vi "main.vi"() -> ()   [LabVIEW 2015]
uses:
  Program Files/C4Utility/c4hdl/win64-x64/LabVIEW/C4Dev_writeFeature.vi
  Program Files/C4Utility/c4hdl/win64-x64/LabVIEW/libC4HdlLV.lvlib
panel:
  in  "camCfg in":string="# simple configuration example of heliInspect H8 using internal motion control\n#\n# Motion parameters in [mm] or [mm/s]\n# exposure ration between 0.0 and 1.0 [1.0 = 100% exposure]\n#\n# enable required components\nComponentSelector = Intensity\nComponentEnable = false\nComponentSelector = Range\nComponentEnable = true\nComponentSelector = Reflectance\nComponentEnable = true\nComponentSelector = Phase\nComponentEnable = false\n#\n# enable required chunk data (optional)\nChunkModeActive = true\nChunkSelector = PartCount\nChunkEnable = true\nChunkSelector = PartType\nChunkEnable = true\n#\n# trigger configuration\nTriggerSelector = RecordingStart\nTriggerMode = On\nTriggerSource = Stage\nTriggerSelector = AcquisitionStart\nTriggerMode = Off\nTriggerSelector = FrameStart\nTriggerMode = On\nTriggerSource = Software\n# Hint: The TriggerSource also controls the TriggerSoftware feature.\n#\n# encoder configuration\nEncoderSelector = Camera\nEncoderInverter = true\n#\n# motion and position configuration\nScanPosition = -1.4\nScanRange = 0.5\nScanSpeed = 5.0\nGeneralSpeed = 10.0\n#\nScanMode = Down\nStageInit = 1\n#\n# additional camera and processing configuration\nScan3dExtractionMethod = AcceleratedCenterOfMassIQCorrection\nScan3dScalingMethod = zTags\nScan3dDistanceUnit = um\n#\nTargetVerticalSpacing = 2.5\nExposureRatio = 1.0\n#\nFPNCorrection = AverageLastFrames\nFPNCorrectionNFrames = 8\nExtSimpMaxHWin = 7\n#\n# illumination control (D3)\nLightControllerSelector = LightController0\nLightControllerSource = UserOutput0\nLightBrightness = 100.0\n# illumination control (D2)\n# LineSelector = Line2\n# LineSource = UserOutput0\n# LineInverter = True\n# switch on the illumination (D2/D3)\nUserOutputSelector = UserOutput0\nUserOutputValue = true"
  out "acqItr":i32
  out "Surface out":dbl[][](graph)
  out "error out":errorcluster
  out "devName out":string[](array[string])
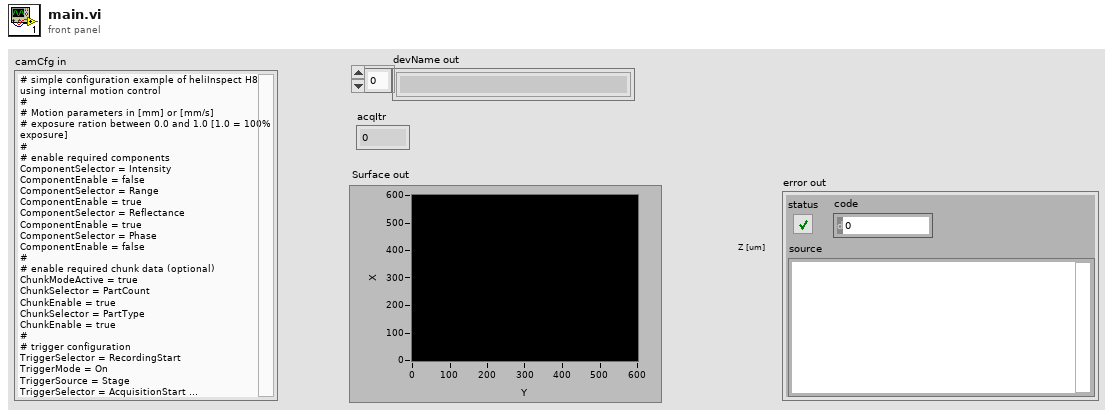
[diagram p1: front panel]
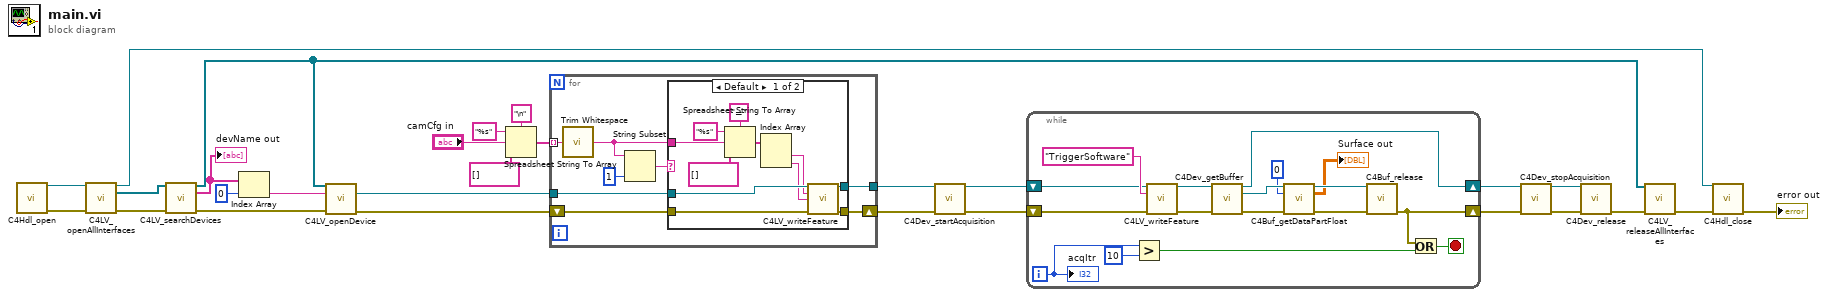
[diagram p0: block diagram]
diagram:
  n1 = call "C4Hdl_open.vi"() -> ("c4hdl out"=w26:refnum<k24>, "error out"=w27:errorcluster)  [unwired: 14 in]
  n2 = call "C4LV_openAllInterfaces.vi"("c4hdl in"=w26, "error in (no error)"=w27) -> ("c4hdl out"=w1:refnum<k24>, "c4if Arr out"=w24:refnum<k24>[], "error out"=w25:errorcluster)  [unwired: 11 in]
  n3 = call "C4LV_searchDevices.vi"("c4if Arr in"=w24, "error in (no error)"=w25) -> ("c4if Arr out"=w11:refnum<k24>[], "devName out"=w23:string[], "error out"=w22:errorcluster)  [unwired: 11 in]
  "devName out" <- w23
  n4 = Index Array(array=w23, index=0) -> (element=w21:string)
  n5 = call "C4LV_openDevice.vi"("c4if Arr in"=w11, "devName in"=w21, "error in (no error)"=w22) -> ("c4dev out"=w20:refnum<k24>, "error out"=w19:errorcluster)  [unwired: 10 in, 1 out]
  n6 = Spreadsheet String To Array(delimiter (Tab)="\n", format string="%s", spreadsheet string="camCfg in", array type (2D Dbl)=string[] [] ("Array Constant")) -> (array=w4:string[])
  n7 = for {
    tunnel: w4 -> [w32] mode=indexing
    tunnel: w20 -> [w33]
    shift-right: [w35] -> w18
    shift-left: w19 -> [w36]
    tunnel: [w34] -> w17
    n8 = call <vilib>:"Trim Whitespace.vi"("string"=w32) -> ("trimmed string"=w31:string)  [unwired: 1 in]
    n9 = String Subset(string=w31, length (rest)=1 ("length (rest)")) -> (substring=w30:string)  [unwired: 1 in]
    n10 = case shown="Default" w30 {
      tunnel: w36 -> [w47 w49]
      tunnel: [w46 w49] -> w35
      tunnel: [w45 w48] -> w34
      tunnel: w33 -> [w44 w48]
      tunnel: w31 -> [w39 _]
      frame Default {
        n11 = Spreadsheet String To Array(delimiter (Tab)="=", format string="%s", spreadsheet string=w39, array type (2D Dbl)=string[] [] ("Array Constant")) -> (array=w43:string[])
        n12 = Index Array(array=w43) -> (element #1=w37:string, element #2=w38:string)  [unwired: 2 in]
        n13 = call-poly "C4LV_writeFeature.vi"("c4dev in"=w44, "name in"=w37, "value in"=w38, "error in"=w47) -> ("c4dev out"=w45:refnum<k24>, "error out"=w46:errorcluster)  [unwired: 10 in]
      }
      frame "#" {
        # "# is a comment"
      }
    }
  }
  n14 = call "C4Dev_startAcquisition.vi"("c4dev in"=w17, "error in (no error)"=w18) -> ("c4dev out"=w16:refnum<k24>, "error out"=w15:errorcluster)  [unwired: 12 in]
  n15 = while {
    shift-right: [w55] -> w10
    shift-left: w15 -> [w56]
    shift-right: [w50] -> w9
    shift-left: w16 -> [w53]
    i -> [w66]
    stop <- w63 stop-if-true
    n16 = Greater?(x=w66, y=10) -> (0:w64:bool)
    n17 = call-poly "C4LV_writeFeature.vi"("c4dev in"=w53, "name in"="TriggerSoftware", "error in"=w56) -> ("c4dev out"=w62:refnum<k24>, "error out"=w57:errorcluster)  [unwired: 11 in]
    n18 = call "C4Dev_getBuffer.vi"("c4dev in"=w62, "error in (no error)"=w57) -> ("c4dev out"=w50:refnum<k24>, "c4buf out"=w60:refnum<k24>, "error out"=w58:errorcluster)  [unwired: 11 in]
    n19 = call "C4Buf_getDataPartFloat.vi"("c4buf in"=w60, "partIdx in"=i64 0, "error in (no error)"=w58) -> ("c4buf out"=w61:refnum<k24>, "data out"=→"Surface out":dbl[][], "error out"=w59:errorcluster)  [unwired: 10 in]
    n20 = call "C4Buf_release.vi"("c4buf in"=w61, "error in (no error)"=w59) -> ("error out"=w55:errorcluster)  [unwired: 13 in]
    n21 = Or(x=w55, y=w64) -> (x .or. y?=w63:bool)
    "acqItr" <- w66
  }
  n22 = call "C4Dev_stopAcquisition.vi"("c4dev in"=w9, "error in (no error)"=w10) -> ("c4dev out"=w13:refnum<k24>, "error out"=w14:errorcluster)  [unwired: 12 in]
  n23 = call "C4Dev_release.vi"("c4dev in"=w13, "error in (no error)"=w14) -> ("error out"=w12:errorcluster)  [unwired: 13 in]
  n24 = call "C4LV_releaseAllInterfaces.vi"("c4if Arr in"=w11, "error in (no error)"=w12) -> ("error out"=w3:errorcluster)  [unwired: 13 in]
  n25 = call "C4Hdl_close.vi"("c4hdl in"=w1, "error in (no error)"=w3) -> ("error out"=→"error out":errorcluster)  [unwired: 13 in]
